vi "SRV_Close TCP Connection.vi"(6 "Force Reset? (F)":bool, 8 "error in":errorcluster, 11 "connection ID":refnum<k5>) -> (0 "error out":errorcluster)   [LabVIEW 2009]
doc: "Closes the SRV connection.\n\n\nModified for Benilde St. Margaret's School - Tim Jump\nBy Doug Schmertman - Logic PD\nCopyright 2012"
uses:
  SubVIs/SRVGlobals.vi
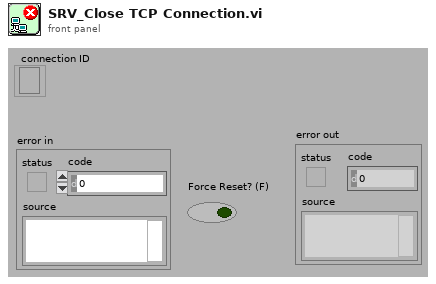
[diagram p1: front panel]
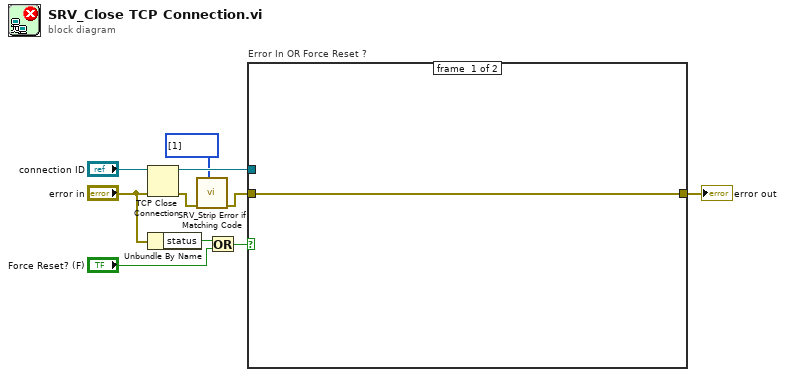
[diagram p0: block diagram]
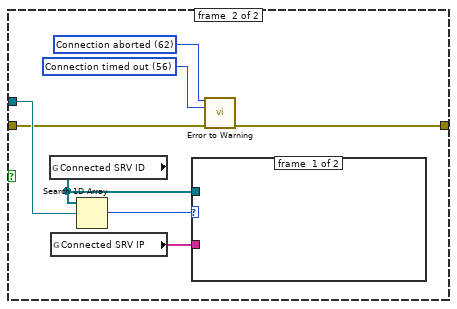
[diagram p2: hidden frame]
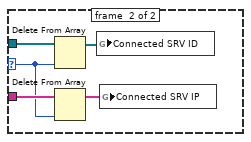
[diagram p3: hidden frame]
diagram:
  n1 = TCP Close Connection(connection ID="connection ID", error in (no error)="error in") -> (connection ID out=w6:refnum<k5>, error out=w3:errorcluster)  [unwired: 1 in]
  n2 = Unbundle By Name("error in") -> ("status"=w9:bool)
  n3 = call "SRV_Strip Error if Matching Code.vi"("error in (no error)"=w3, "Strip Codes"=i32[] [1]) -> ("error out"=w2:errorcluster)  [unwired: 8 in]
  n4 = Or(x=w9, y="Force Reset? (F)") -> (x .or. y?=w7:bool)
  n5 = case "Error In OR Force Reset ?" shown="True" w7 {
    tunnel: w6 -> [_ w16]
    tunnel: [w11 w17] -> w10
    tunnel: w2 -> [w11 w12]
    frame #0 {
    }
    frame #1 {
      w19 = 56 items=["No Error", "Argument Error", "Memory Full", "Out of Zone", "End of File", "File Already Open", "Generic File IO Error", "File Not Found", "File Permission Error", "Disk Full", "Duplicate Path", "Too Many Files Open", "Not Enabled", "Resource File Not Found", "Cannot Add Resource", "Resource Not Found", "Image Not Found", "Image Memory Error", "Pen Does Not Exist", "Config Bad Type", "Config Token Not Found", "Config Parse Error", "Config Memory Error", "Bad External Code Format", "Bad External Code Offset", "External Code Not Present", "Null Window", "Destroy Window Mixup", "Null Menu", "Print Aborted", "Bad Print Record", "Print Driver Error", "Windows Error During Print", "Memory Error During Print", "Print Dialog Error", "Generic Print Error", "Invalid Device Refnum", "Device Not Found", "Device Parameter Error", "Device Unit Error", "Can't Open Device", "Device Call Aborted", "Generic Error", "Cancelled By User", "Object ID Too Low", "Object ID Too High", "Object Not In Heap", "Unknown Heap", "Bad DefProc ID", "DefProc Not In Table", "Message Out Of Range", "Null Method", "Unknown Message", "Manager Call Not Supported", "Bad address", "Connection In progress", "Connection timed out", "Connection is already in progress", "Network attribute not supported", "Network error", "Address in use", "System out of memory", "Connection aborted", "Connection refused", "Connection is not connected", "Connection is already connected", "Connection closed", "Initialize error (interapplication manager)", "Bad occurrence", "Wait on unbound occurrence handler", "Occurrence queue overflow", "Bad path", "Semaphore not signaled", "Unrecognized type (interapplication manager)"] ("2nd Error to Convert")
      w18 = 62 items=["No Error", "Argument Error", "Memory Full", "Out of Zone", "End of File", "File Already Open", "Generic File IO Error", "File Not Found", "File Permission Error", "Disk Full", "Duplicate Path", "Too Many Files Open", "Not Enabled", "Resource File Not Found", "Cannot Add Resource", "Resource Not Found", "Image Not Found", "Image Memory Error", "Pen Does Not Exist", "Config Bad Type", "Config Token Not Found", "Config Parse Error", "Config Memory Error", "Bad External Code Format", "Bad External Code Offset", "External Code Not Present", "Null Window", "Destroy Window Mixup", "Null Menu", "Print Aborted", "Bad Print Record", "Print Driver Error", "Windows Error During Print", "Memory Error During Print", "Print Dialog Error", "Generic Print Error", "Invalid Device Refnum", "Device Not Found", "Device Parameter Error", "Device Unit Error", "Can't Open Device", "Device Call Aborted", "Generic Error", "Cancelled By User", "Object ID Too Low", "Object ID Too High", "Object Not In Heap", "Unknown Heap", "Bad DefProc ID", "DefProc Not In Table", "Message Out Of Range", "Null Method", "Unknown Message", "Manager Call Not Supported", "Bad address", "Connection In progress", "Connection timed out", "Connection is already in progress", "Network attribute not supported", "Network error", "Address in use", "System out of memory", "Connection aborted", "Connection refused", "Connection is not connected", "Connection is already connected", "Connection closed", "Initialize error (interapplication manager)", "Bad occurrence", "Wait on unbound occurrence handler", "Occurrence queue overflow", "Bad path", "Semaphore not signaled", "Unrecognized type (interapplication manager)"] ("1st Error to Convert")
      n6 = global read "SRVGlobals.vi" "Connected SRV ID"() -> (w15:refnum<k5>[])
      n7 = global read "SRVGlobals.vi" "Connected SRV IP"() -> (w14:string[])
      n8 = Search 1D Array(1D array=w15, element=w16) -> (index of element=w13:i32)  [unwired: 1 in]
      n9 = case shown="Default" w13 {
        selector: w13 -> [_ w20]
        tunnel: w15 -> [_ w24]
        tunnel: w14 -> [_ w23]
        frame #0 {
        }
        frame #1 {
          n10 = Delete From Array(array=w24, index=w20) -> (array with subset deleted=w21:refnum<k5>[])  [unwired: 1 in, 1 out]
          n11 = Delete From Array(array=w23, index=w20) -> (array with subset deleted=w22:string[])  [unwired: 1 in, 1 out]
          n12 = global write "SRVGlobals.vi" "Connected SRV ID"(w21) -> ()
          n13 = global write "SRVGlobals.vi" "Connected SRV IP"(w22) -> ()
        }
      }
      n14 = call <vilib>:"Error to Warning.vi"("1st Error to Convert"=w18, "2nd Error to Convert"=w19, "error in"=w12) -> ("warning out"=w17:errorcluster)  [unwired: 12 in]
    }
  }
  "error out" <- w10
